vi "SetupDataSet.vi"(10 "字符串":string) -> (2 "item data":string)   [LabVIEW 2018]
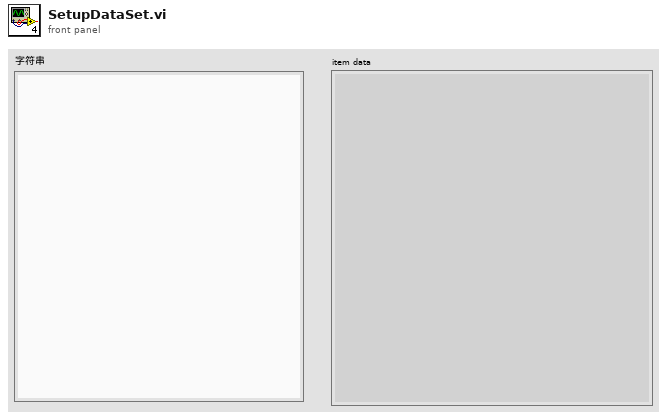
[diagram p1: front panel]
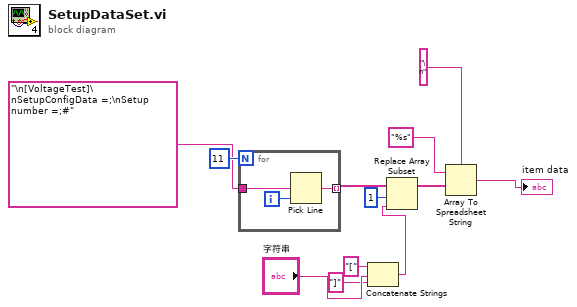
[diagram p0: block diagram]
diagram:
  n1 = for {
    N: 11 -> [_]
    tunnel: "\n[VoltageTest]\nSetupConfigData =;\nSetup number =;#" -> [w14]
    tunnel: [w15] -> w3 mode=indexing
    i -> [w13]
    n2 = Pick Line(multi-line string=w14, line index=w13) -> (output string=w15:string)  [unwired: 1 in]
  }
  n3 = Concatenate Strings("[" ("字符串"), "字符串", "]" ("字符串")) -> (w10:string)
  n4 = Replace Array Subset(array=w3, new element=w10, index=1 ("索引")) -> (w4:string[])
  n5 = Array To Spreadsheet String(delimiter (Tab)="\n" ("分隔符(Tab)"), array=w4, 3:"%s" ("格式字符串")) -> (spreadsheet string=→"item data":string)
